vi "Add Alias_Alias Internal_Alias and Folders.vi"(8 "error in (no error)":errorcluster, 9 "Alias Settings":T1, 11 "Alias Ref":refnum<k24>) -> (0 "error out":errorcluster, 3 "Alias Ref Out":refnum<k24>)   [LabVIEW 2019, in "Simple SysDef API.lvlib"]
uses:
  <userlib>/SimpleSysDef/Simple SysDef API.lvlib
  NationalInstruments.VeriStand.SystemDefinitionAPI
  <userlib>/SimpleSysDef/_SubVIs/Add Alias_Alias Settings.ctl
  <userlib>/SimpleSysDef/_SubVIs/Add Folder_Settings.ctl
  <vilib>/Utility/error.llb/Trim Whitespace One-Sided.vi
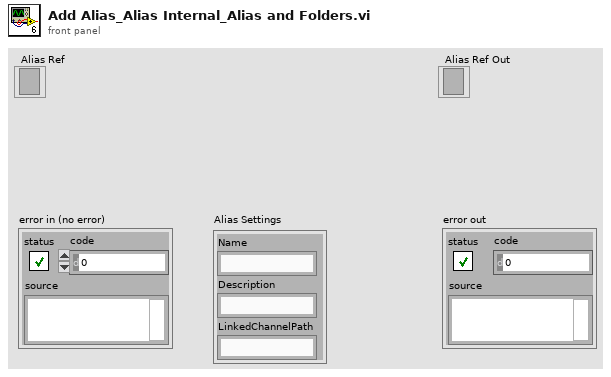
[diagram p1: front panel]
types:
  T1 = typedef "Simple SysDef API.lvlib/Add Alias_Alias Settings.ctl" = cluster{"Name":string, "Description":string, "LinkedChannelPath":string}
  T2 = typedef "Simple SysDef API.lvlib/Add Folder_Settings.ctl" = cluster{"Name":string, "Description":string}
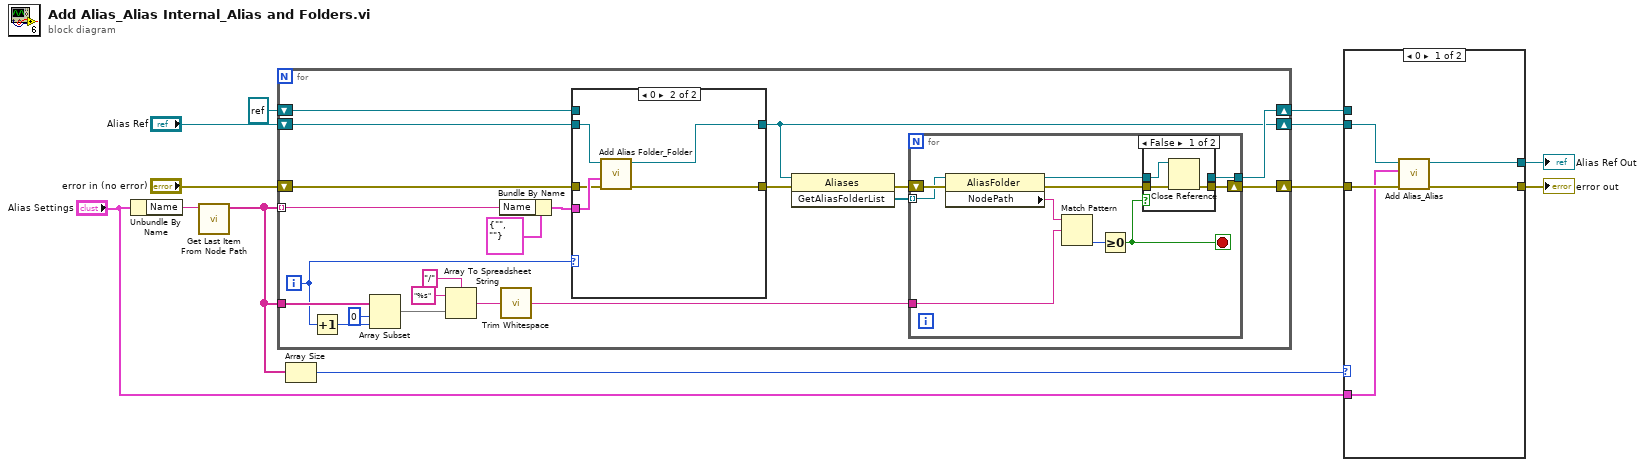
[diagram p0: block diagram]
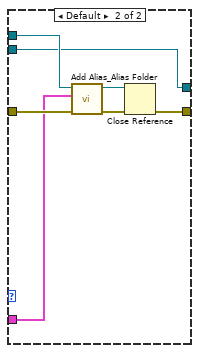
[diagram p2: hidden frame]
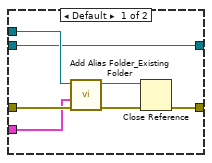
[diagram p4: hidden frame]
diagram:
  n1 = Unbundle By Name("Alias Settings") -> ("Name"=w5:string)
  n2 = call <userlib>:"Get Last Item From Node Path.vi"("Name"=w5) -> ("First Items"=w10:string[])  [unwired: 9 in, 1 out]
  n3 = for {
    tunnel: w10 -> [w30] mode=indexing
    shift-right: [w16] -> w8
    shift-left: "error in (no error)" -> [w31]
    shift-right: [w17] -> w7
    shift-left: refnum<k24> refnum -> [w29]
    tunnel: w10 -> [w28]
    shift-right: [w13] -> w6
    shift-left: "Alias Ref" -> [w14]
    i -> [w27]
    n4 = Increment(x=w27) -> (x+1=w26:i32)
    n5 = Array Subset(array=w28, index=0, length=w26) -> (w24:string[])
    n6 = Array To Spreadsheet String(delimiter (Tab)="/", array=w24, 3:"%s" ("format string")) -> (spreadsheet string=w21:string)
    n7 = Bundle By Name(cluster=T2 {"Name"="", "Description"=""} ("Alias Folder Settings"), "Name"=w30) -> (w32:T2)
    n8 = call <vilib>:"Trim Whitespace.vi"("string"=w21) -> ("trimmed string"=w15:string)  [unwired: 1 in]
    n9 = case shown="0" w27 {
      tunnel: w14 -> [w52 w60]
      tunnel: w32 -> [w53 w59]
      tunnel: w31 -> [w54 w58]
      tunnel: w29 -> [w55 _]
      tunnel: [w49 w57] -> w18
      tunnel: [w52 w56] -> w13
      frame Default {
        n10 = call <userlib>:"Add Alias Folder_Existing Folder.vi"("error in (no error)"=w54, "Alias Folder Settings"=w53, "Alias Folder Ref"=w55) -> ("error out"=w50:errorcluster, "Alias Folder Ref out"=w51:refnum<k24>)  [unwired: 7 in]
        n11 = Close Reference(reference=w51, error in (no error)=w50) -> (error out=w49:errorcluster)
      }
      frame 0 {
        n12 = call <userlib>:"Add Alias Folder_Folder.vi"("error in (no error)"=w58, "Alias Folder Settings"=w59, "Alias Folder Ref"=w60) -> ("error out"=w57:errorcluster, "Alias Folder Ref out"=w56:refnum<k24>)  [unwired: 7 in]
      }
    }
    n13 = invoke class="Aliases" method="GetAliasFolderList"(reference=w13, error in=w18) -> (error out=w20:errorcluster, "GetAliasFolderList"=w19:refnum<k24>[])  [unwired: 1 in, 1 out]
    n14 = for {
      shift-right: [w36] -> w16
      shift-left: w20 -> [w43]
      tunnel: w19 -> [w42] mode=indexing
      tunnel: w15 -> [w40]
      tunnel: [w35] -> w17
      stop <- w34 stop-if-true
      n15 = property class="AliasFolder"(reference=w42, error in=w43) -> (reference out=w37:refnum<k24>, error out=w38:errorcluster, "NodePath"=w41:string)
      n16 = Match Pattern(string=w41, regular expression=w40) -> (offset past match=w39:i32)  [unwired: 1 in, 3 out]
      n17 = Greater Or Equal To 0?(x=w39) -> (x >= 0?=w34:bool)
      n18 = case shown="False" w34 {
        tunnel: w38 -> [w46 w47]
        tunnel: w37 -> [w45 w48]
        tunnel: [w44 w47] -> w36
        tunnel: [_ w48] -> w35
        frame False {
          n19 = Close Reference(reference=w45, error in (no error)=w46) -> (error out=w44:errorcluster)
        }
        frame True {
        }
      }
    }
  }
  n20 = Array Size(array=w10) -> (size(s)=w9:i32)
  n21 = case shown="0" w9 {
    tunnel: w8 -> [w65 w72]
    tunnel: w7 -> [_ w71]
    tunnel: w6 -> [w64 w66]
    tunnel: [w63 w68] -> w3
    tunnel: "Alias Settings" -> [w62 w70]
    tunnel: [w61 w66] -> w2
    frame 0 {
      n22 = call <userlib>:"Add Alias_Alias.vi"("error in (no error)"=w65, "Alias Settings"=w62, "Aliases Ref"=w64) -> ("error out"=w63:errorcluster, "Aliases Ref Out"=w61:refnum<k24>)  [unwired: 7 in]
    }
    frame Default {
      n23 = call <userlib>:"Add Alias_Alias Folder.vi"("error in (no error)"=w72, "Alias Settings"=w70, "Aliases Folder Ref"=w71) -> ("error out"=w69:errorcluster, "Aliases Folder Ref Out"=w67:refnum<k24>)  [unwired: 7 in]
      n24 = Close Reference(reference=w67, error in (no error)=w69) -> (error out=w68:errorcluster)
    }
  }
  "error out" <- w3
  "Alias Ref Out" <- w2
